vi "Data_DisplayInfo.vi"(5 "header size":i32, 9 "file wfm info":T1) -> (8 "回放信息":string)   [LabVIEW 2013]
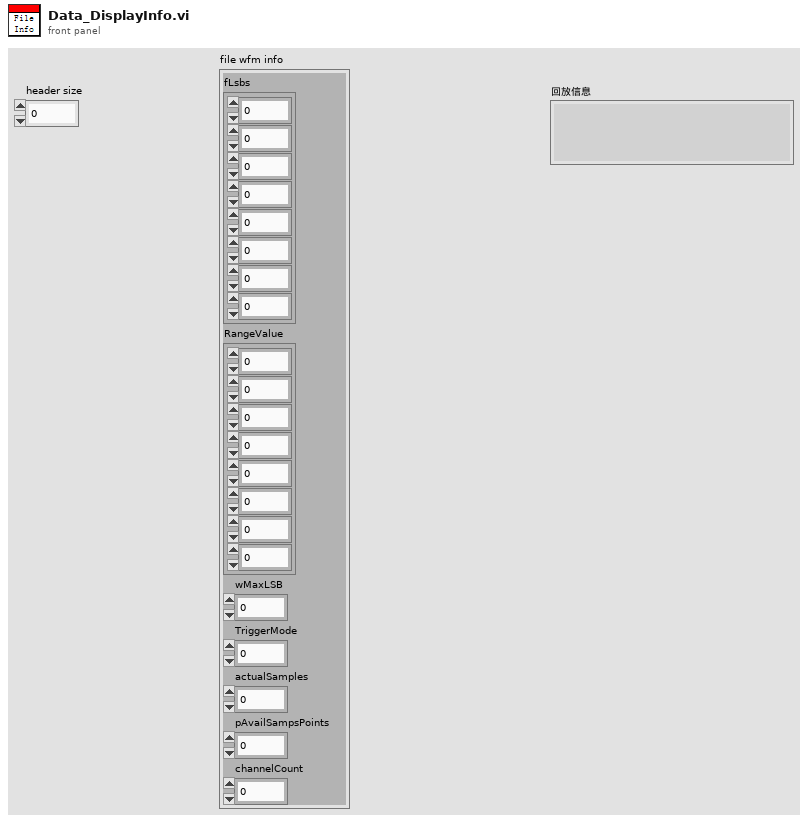
[diagram p1: front panel]
types:
  T1 = cluster{"fLsbs":cluster{dbl, dbl, dbl, dbl, dbl, dbl, dbl, dbl}, "RangeValue":cluster{dbl, dbl, dbl, dbl, dbl, dbl, dbl, dbl}, "wMaxLSB":u32, "TriggerMode":i32, "actualSamples":u32, "pAvailSampsPoints":u32, "channelCount":i32}
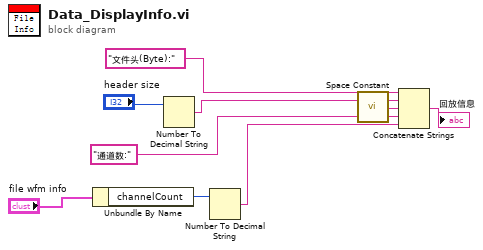
[diagram p0: block diagram]
diagram:
  n1 = Unbundle By Name("file wfm info") -> ("channelCount"=w5:i32)
  n2 = Number To Decimal String(number="header size") -> (decimal integer string=w7:string)  [unwired: 1 in]
  n3 = Number To Decimal String(number=w5) -> (decimal integer string=w3:string)  [unwired: 1 in]
  n4 = call <vilib>:"Space Constant.vi"() -> ("String"=w1:string)
  n5 = Concatenate Strings("文件头(Byte):" ("字符串"), w7, w1, "通道数:" ("字符串"), w3) -> (→"回放信息":string)
